vi "Exit.vi"(8 "Error In":errorcluster, 11 "Model in":refnum<class "Model.lvclass">) -> (0 "Error Out":errorcluster, 3 "Model out":refnum<class "Model.lvclass">)   [LabVIEW 2021, in "Model.lvclass"]
doc: "This VI closes the VI reference of Analog to Digital Convertor VI and stops the running VI."
uses:
  Model.lvclass
  Controls/Queue Operation.ctl
  Controls/State Cluster.ctl
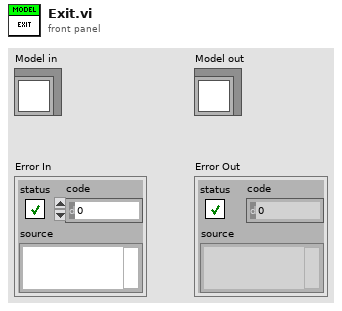
[diagram p1: front panel]
types:
  T1 = typedef "State Cluster.ctl" = cluster{"State":string, "Data":variant}
  T2 = typedef "Queue Operation.ctl" = enum16{"Create", "Enqueue", "Enqueue N", "Enstack", "Dequeue", "Flush", "Release"}
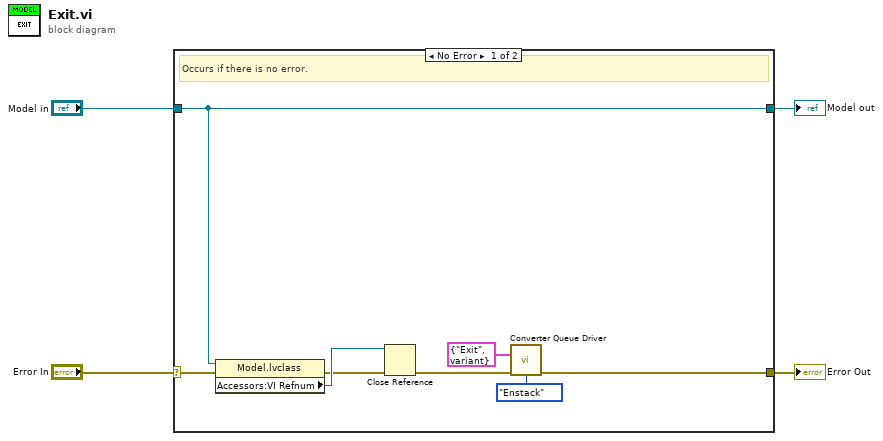
[diagram p0: block diagram]
diagram:
  n1 = case shown="No Error" "Error In" {
    selector: "Error In" -> [w12 w14]
    tunnel: [w5 w14] -> w3
    tunnel: [w9 w13] -> w1
    tunnel: "Model in" -> [w9 w13]
    frame No Error {
      # "Occurs if there is no error."
      n2 = property class="Model.lvclass"(reference=w9, error in=w12) -> (error out=w7:errorcluster, "Accessors:VI Refnum"=w8:refnum<vi>)  [unwired: 1 out]
      n3 = Close Reference(reference=w8, error in (no error)=w7) -> (error out=w6:errorcluster)
      n4 = call "Converter Queue Driver.vi"("State"=T1 {"State"="Exit", "Data"=variant}, "error in (no error)"=w6, "Operation"=Queue_Operation."Enstack") -> ("error out"=w5:errorcluster)  [unwired: 11 in, 1 out]
    }
    frame Error {
      # "Occurs if there is any error."
    }
  }
  "Error Out" <- w3
  "Model out" <- w1
